vi "Weather Station UI.vi"() -> ()   [LabVIEW 2014]
doc: "이 VI는 Weather Station 프로젝트의 Main VI입니다. 이 VI에는 온도 경고 시스템의 사용자 인터페이스가 들어있습니다. 매 .5초마다 온도가 수집됩니다; 경고가 발생하면 데이터가 로그됩니다."
uses:
  Instance           2 26Saved   Weather Station UI .vi
panel:
  out "경고":string
  in  "하위 리미트":dbl=20.0
  in  "상위 리미트":dbl=30.0
  in  "정지 버튼":bool
  out "온도 히스토리":dbl(graph)
  # "온도 범위(C)"
  # "동상"
  # "열사병"
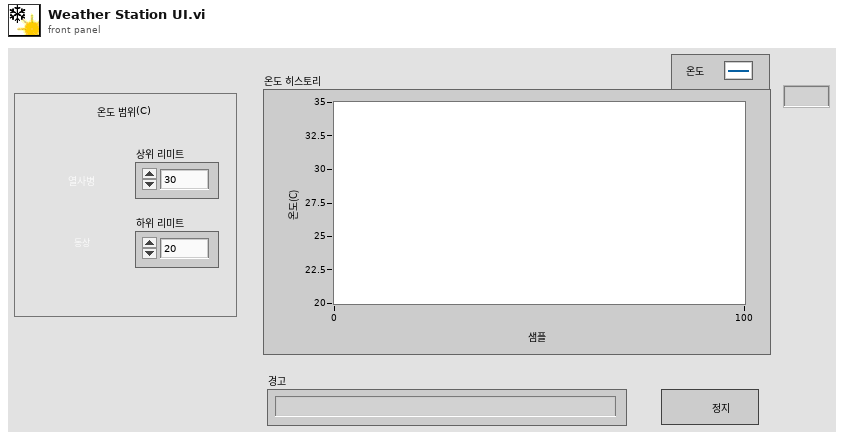
[diagram p1: front panel]
types:
  T1 = enum16{"open", "replace", "create", "open or create", "replace or create", "replace or create with confirmation"}
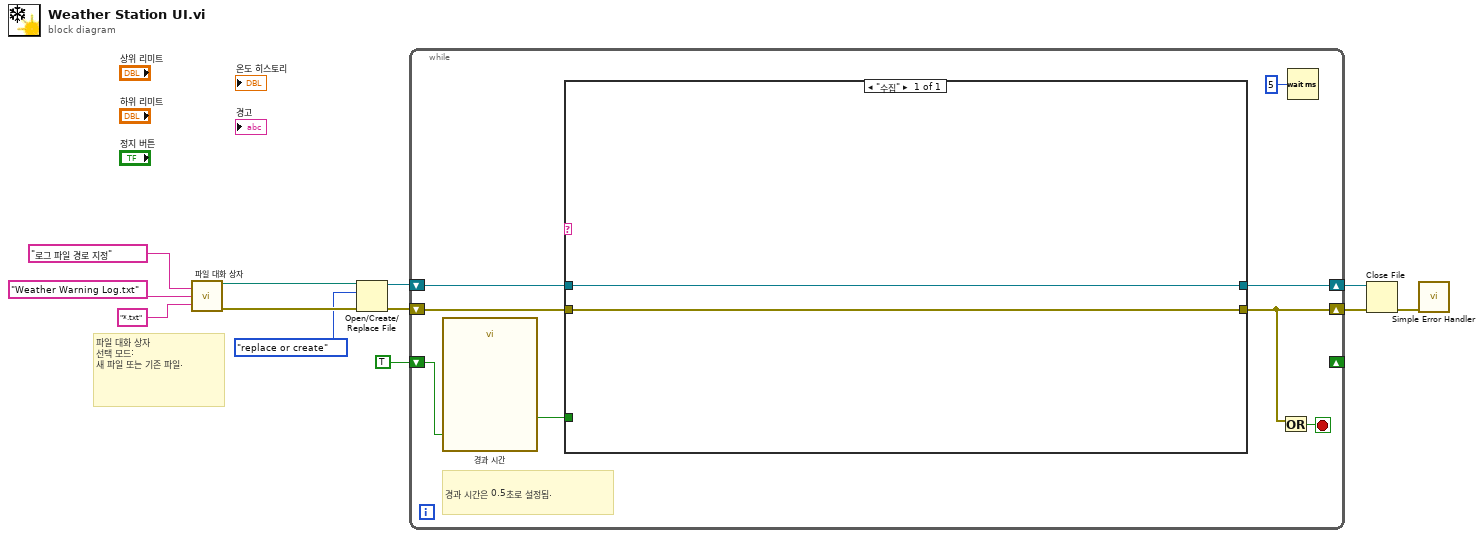
[diagram p0: block diagram]
diagram:
  # "파일 대화 상자\n선택 모드:\n새 파일 또는 기존 파일."
  n1 = call "파일 대화 상자"("prompt"="로그 파일 경로 지정" ("입력 요청"), "default name"="Weather Warning Log.txt" ("기본 이름"), "pattern (all files)"="*.txt" ("패턴 라벨")) -> ("selected path"=w6:path, "error out"=w3:errorcluster)  [unwired: 9 in, 2 out]
  n2 = Open/Create/Replace File(file path (use dialog)=w6, error in=w3, operation (0:open)=T1."replace or create" ("동작 (0:열기)")) -> (refnum out=w8:refnum<file>, error out=w7:errorcluster)  [unwired: 3 in, 1 out]
  n3 = while {
    shift-right: [w13] -> w12
    shift-left: w7 -> [w20]
    shift-right: [w18] -> w11
    shift-left: w8 -> [w17]
    shift-right: _ -> [_]
    shift-left: TRUE ("정지") -> [w15]
    stop <- w19 stop-if-true
    # "경과 시간은 0.5초로 설정됨."
    n4 = call "경과 시간"("Reset"=w15) -> ("Time has Elapsed"=w14:bool)  [unwired: 11 in, 7 out]
    n5 = case shown="\"수집\"" {
      selector: _ -> [_]
      tunnel: [w21] -> w13
      tunnel: w20 -> [w21]
      tunnel: [w22] -> w18
      tunnel: w17 -> [w22]
      tunnel: w14 -> [_]
      frame "수집" {
      }
    }
    n6 = Or(x=w13) -> (x .or. y?=w19:bool)  [unwired: 1 in]
    n7 = Wait (ms)(milliseconds to wait=u32 5 ("y")) -> ()  [unwired: 1 out]
  }
  n8 = Close File(refnum=w11, error in=w12) -> (error out=w10:errorcluster)  [unwired: 1 out]
  n9 = call <vilib>:"Simple Error Handler.vi"("error in (no error)"=w10) -> ()  [unwired: 4 in, 5 out]
